vi "CameraControl.vi"(0 "Exposure Time":dbl=20011.0 min=61.0 max=16000000.0, 1 "Gain Selector":u32(ring)=1 items=["Sensor", "Digital"], 2 "Gain":dbl=1.0 min=1.0 max=4.0, 3 "Gain (Raw)":i64 min=0 max=384 step=1, 4 "Black Level Selector":u32(ring) items=["Analog"], 5 "Stop (F)":bool, 7 "error in":errorcluster, 8 "Black Level":dbl=240.0 min=0.0 max=511.0, 9 "Camera":string="S1104113") -> (6 "Lost Packet Count":u32, 20 "Image Out":T1(plugin-control), 21 "All Image Buffers Out":T1[](array[typedef]), 22 "Temp":dbl, 26 "Stopped":bool, 27 "error out":errorcluster)   [LabVIEW 2014]
doc: "Creates, and edits acquisitions using the NI Vision Acquisition Express VI.\n\nThe NI Vision Acquisition Wizard is launched by placing the Express VI on the block diagram. Select an acquisition source and configure an acquisition using NI-IMAQ, NI-IMAQdx, or simulate an acquisition by reading an AVI or image files from a folder. After an acquisition is configured, select controls and indicators to be able to programmatically set in LabVIEW. Double-click the Vision Acquisition Express VI to edit the acquisition.\n\nNote: Any images created by the Express VI need to be disposed after use. Use the IMAQ Dispose.vi to cleanup the images output by the Express VI when they are no longer needed."
uses:
  <vilib>/vision/Image Controls.llb/IMAQ Image.ctl
  <vilib>/vision/driver/IMAQdx.llb/IMAQdx Buffer Number Mode.ctl
  <vilib>/vision/driver/NI_Vision_Acquisition_Software.lvlib
  <resource>/objmgr/imaqdx.rc
panel:
  out "BufferCount":u32
  out "LostBufferCount":u32
  out "x != y? 6":bool
  out "x != y? 5":bool
  out "x != y? 4":bool
  out "x != y? 3":bool
  out "x != y? 2":bool
  out "x != y?":bool
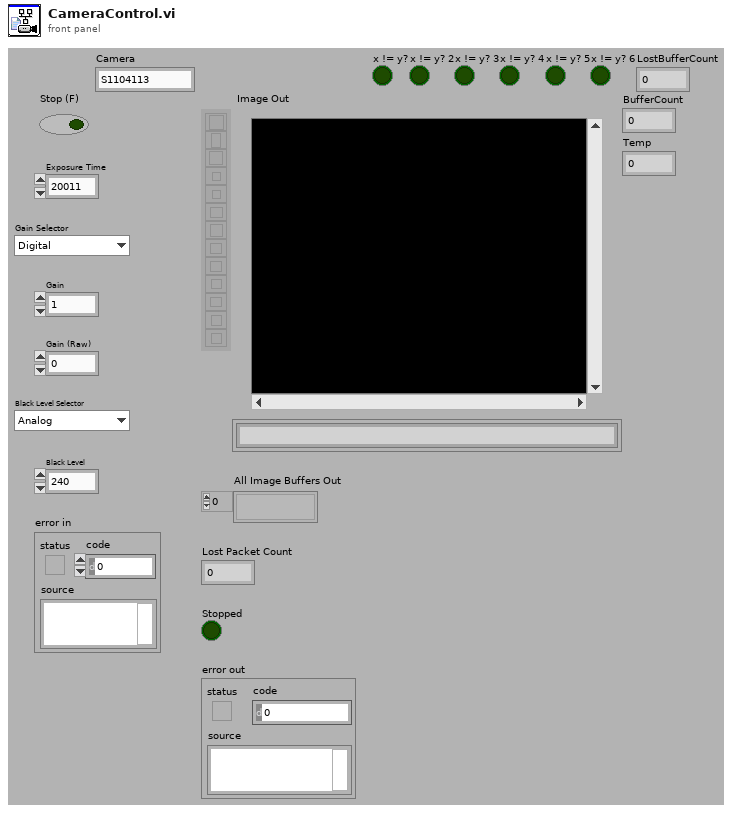
[diagram p1: front panel]
types:
  T1 = typedef "IMAQ Image.ctl" = refnum<image>
  T2 = typedef "NI_Vision_Acquisition_Software.lvlib/IMAQdx Buffer Number Mode.ctl" = enum32{"Next", "Last", "Buffer Number"}
  T3 = typedef "IMAQdx.ctl" = refnum<k21>
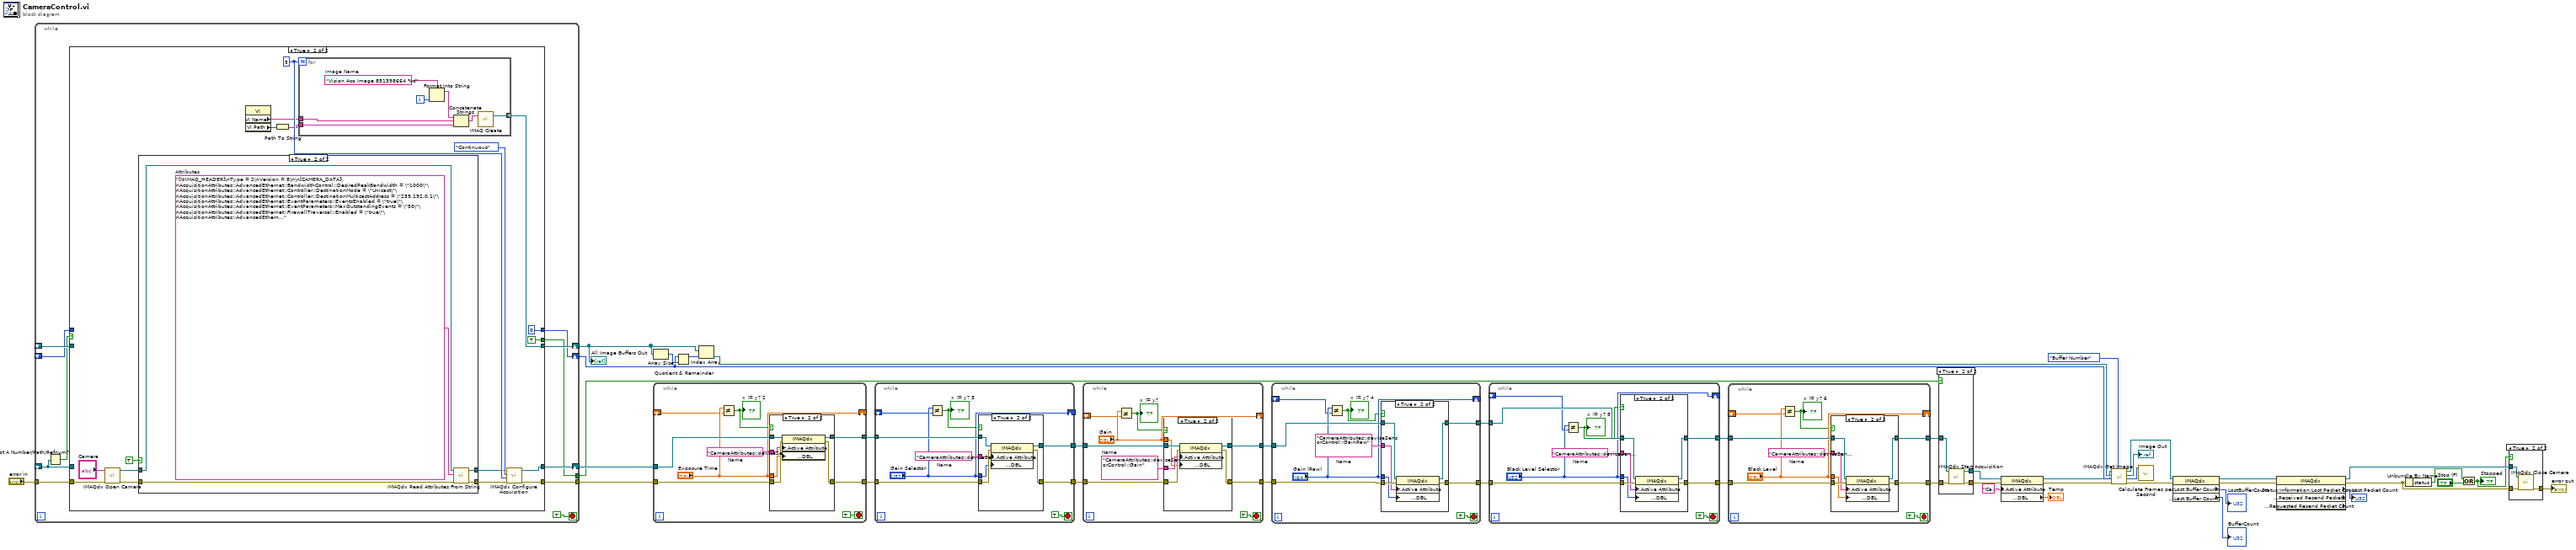
[diagram p0: block diagram]
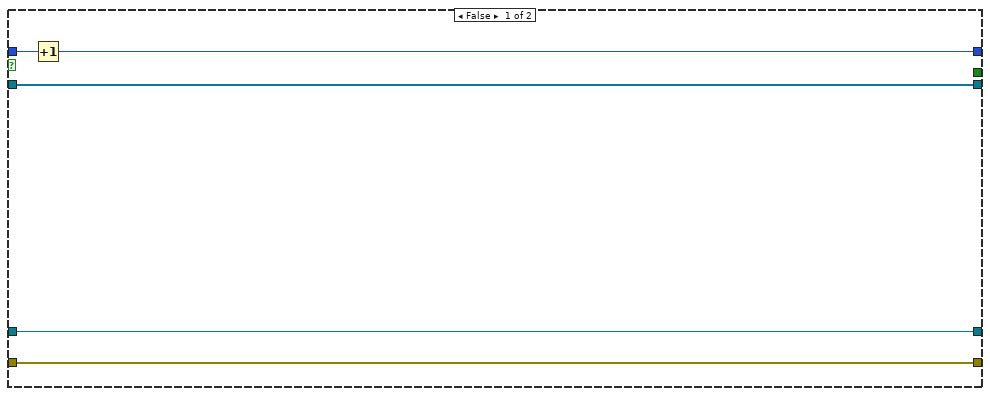
[diagram p10: hidden frame]
diagram:
  n1 = while {
    shift-right: [w54] -> w41
    shift-left: _ -> [w46]
    tunnel: [w53] -> w42
    tunnel: "error in" -> [w52]
    shift-right: [w50] -> w26
    shift-left: _ -> [w49]
    shift-right: [w48] -> w21
    shift-left: _ -> [w47]
    tunnel: [w44] -> w20
    stop <- TRUE stop-if-true
    n2 = Not A Number/Path/Refnum?(number/path/refnum=w46) -> (NaN/Path/Refnum?=w45:bool)
    n3 = case shown="True" w45 {
      tunnel: [w59 w60] -> w54
      tunnel: w46 -> [w59 _]
      tunnel: [w58 w75] -> w53
      tunnel: w52 -> [w58 w76]
      tunnel: [w57 w74] -> w50
      tunnel: w49 -> [w57 _]
      tunnel: [w55 0] -> w48
      tunnel: w47 -> [w56 _]
      tunnel: [_ TRUE] -> w44
      frame False {
        n4 = Increment(x=w56) -> (x+1=w55:i32)
      }
      frame True {
        w73 = u32 5 ("Number of Image Buffers")
        n5 = call <vilib>:"IMAQdx Open Camera.vi"("error in"=w76, "Session In"="Camera") -> ("error out"=w66:errorcluster, "Session Out"=w67:T3)  [unwired: 1 in, 7 out]
        n6 = case shown="True" TRUE ("Init Attributes") {
          tunnel: w67 -> [w78 w83]
          tunnel: w66 -> [w77 w82]
          tunnel: [w78 w79] -> w65
          tunnel: [w77 w80] -> w64
          frame False {
          }
          frame True {
            w81 = "[NIIMAQ_HEADER]\nType = 2\nVersion = 8\n\n[CAMERA_DATA]\nAcquisitionAttributes::AdvancedEthernet::BandwidthControl::DesiredPeakBandwidth = \"1000\"\nAcquisitionAttributes::AdvancedEthernet::Controller::DestinationMode = \"Unicast\"\nAcquisitionAttributes::AdvancedEthernet::Controller::DestinationMulticastAddress = \"239.192.0.1\"\nAcquisitionAttributes::AdvancedEthernet::EventParameters::EventsEnabled = \"true\"\nAcquisitionAttributes::AdvancedEthernet::EventParameters::MaxOutstandingEvents = \"50\"\nAcquisitionAttributes::AdvancedEthernet::FirewallTraversal::Enabled = \"true\"\nAcquisitionAttributes::AdvancedEthernet::FirewallTraversal::KeepAliveTime = \"30\"\nAcquisitionAttributes::AdvancedEthernet::ResendParameters::MaxResendsPerPacket = \"25\"\nAcquisitionAttributes::AdvancedEthernet::ResendParameters::MemoryWindowSize = \"1024\"\nAcquisitionAttributes::AdvancedEthernet::ResendParameters::MissingPacketTimeout = \"2\"\nAcquisitionAttributes::AdvancedEthernet::ResendParameters::NewPacketTimeout = \"100\"\nAcquisitionAttributes::AdvancedEthernet::ResendParameters::ResendBatchingPercentage = \"10\"\nAcquisitionAttributes::AdvancedEthernet::ResendParameters::ResendResponseTimeout = \"2\"\nAcquisitionAttributes::AdvancedEthernet::ResendParameters::ResendsEnabled = \"true\"\nAcquisitionAttributes::AdvancedEthernet::ResendParameters::ResendThresholdPercentage = \"5\"\nAcquisitionAttributes::AdvancedEthernet::ResendParameters::ResendTimerResolution = \"1\"\nAcquisitionAttributes::AdvancedEthernet::TestPacketParameters::MaxTestPacketRetries = \"1\"\nAcquisitionAttributes::AdvancedEthernet::TestPacketParameters::TestPacketEnabled = \"true\"\nAcquisitionAttributes::AdvancedEthernet::TestPacketParameters::TestPacketTimeout = \"250\"\nAcquisitionAttributes::AdvancedGenicam::CommandTimeout = \"100\"\nAcquisitionAttributes::Bayer::Algorithm = \"Bilinear\"\nAcquisitionAttributes::Bayer::GainB = \"1\"\nAcquisitionAttributes::Bayer::GainG = \"1\"\nAcquisitionAttributes::Bayer::GainR = \"1\"\nAcquisitionAttributes::Bayer::Pattern = \"Use hardware value\"\nAcquisitionAttributes::BitsPerPixel = \"Use hardware value\"\nAcquisitionAttributes::ChunkDataDecoding::ChunkDataDecodingEnabled = \"false\"\nAcquisitionAttributes::ChunkDataDecoding::MaximumChunkCopySize = \"64\"\nAcquisitionAttributes::IgnoreFirstFrame = \"false\"\nAcquisitionAttributes::ImageDecoderCopyMode = \"Auto\"\nAcquisitionAttributes::IncompleteBufferMode = \"Ignore\"\nAcquisitionAttributes::OutputImageType = \"Auto\"\nAcquisitionAttributes::OverwriteMode = \"Get Newest\"\nAcquisitionAttributes::PacketSize = \"1500\"\nAcquisitionAttributes::PixelSignedness = \"Use hardware value\"\nAcquisitionAttributes::ReceiveTimestampMode = \"None\"\nAcquisitionAttributes::ShiftPixelBits = \"false\"\nAcquisitionAttributes::SwapPixelBytes = \"false\"\nAcquisitionAttributes::Timeout = \"5000\"\nCameraAttributes::deviceCounterAndTimerControl::counterSelector = \"Counter 1\"\nCameraAttributes::deviceCounterAndTimerControl::counterMode = \"Off\"\nCameraAttributes::deviceCounterAndTimerControl::counterStartSource = \"Line 1\"\nCameraAttributes::deviceCounterAndTimerControl::counterStartLineActivation = \"Rising Edge\"\nCameraAttributes::deviceCounterAndTimerControl::counterIncrementalSource = \"Internal Clock\"\nCameraAttributes::deviceCounterAndTimerControl::counterResetSource = \"Reset Cmd\"\nCameraAttributes::deviceCounterAndTimerControl::counterDuration = \"1\"\nCameraAttributes::deviceCounterAndTimerControl::timerSelector = \"Timer 1\"\nCameraAttributes::deviceCounterAndTimerControl::timerMode = \"Off\"\nCameraAttributes::deviceCounterAndTimerControl::timerStartSource = \"Line 1\"\nCameraAttributes::deviceCounterAndTimerControl::timerStartLineActivation = \"Rising Edge\"\nCameraAttributes::deviceCounterAndTimerControl::timerDuration = \"1\"\nCameraAttributes::deviceSensorControl::AcquisitionFrameRate = \"30\"\nCameraAttributes::deviceSensorControl::BlackLevelSelector = \"Analog\"\nCameraAttributes::deviceSensorControl::BlackLevelRaw = \"240\"\nCameraAttributes::deviceSensorControl::exposureAlignment = \"Synchronous\"\nCameraAttributes::deviceSensorControl::ExposureMode = \"Timed\"\nCameraAttributes::deviceSensorControl::ExposureTime = \"20011\"\nCameraAttributes::deviceSensorControl::GainSelector = \"Sensor\"\nCameraAttributes::deviceSensorControl::Gain = \"1\"\nCameraAttributes::deviceSensorControl::GainSelector = \"Digital\"\nCameraAttributes::deviceSensorControl::Gain = \"1\"\nCameraAttributes::DigitalIOControl::LineSelector = \"Line 1\"\nCameraAttributes::DigitalIOControl::lineDetectionLevel = \"Threshold for TTL\"\nCameraAttributes::DigitalIOControl::LineInverter = \"false\"\nCameraAttributes::DigitalIOControl::lineDebouncingPeriod = \"0\"\nCameraAttributes::DigitalIOControl::LineSelector = \"Line 2\"\nCameraAttributes::DigitalIOControl::lineDetectionLevel = \"Threshold for TTL\"\nCameraAttributes::DigitalIOControl::LineInverter = \"false\"\nCameraAttributes::DigitalIOControl::lineDebouncingPeriod = \"0\"\nCameraAttributes::DigitalIOControl::LineSelector = \"Line 3\"\nCameraAttributes::DigitalIOControl::LineInverter = \"false\"\nCameraAttributes::DigitalIOControl::outputLineSource = \"Pulse On: Software Command\"\nCameraAttributes::DigitalIOControl::outputLinePulseDelay = \"0\"\nCameraAttributes::DigitalIOControl::outputLinePulseDuration = \"1\"\nCameraAttributes::DigitalIOControl::LineSelector = \"Line 4\"\nCameraAttributes::DigitalIOControl::LineInverter = \"false\"\nCameraAttributes::DigitalIOControl::outputLineSource = \"Pulse On: Software Command\"\nCameraAttributes::DigitalIOControl::outputLinePulseDelay = \"0\"\nCameraAttributes::DigitalIOControl::outputLinePulseDuration = \"1\"\nCameraAttributes::DigitalIOControl::LineSelector = \"Line 1\"\nCameraAttributes::DigitalIOControl::TriggerSelector = \"Single Frame Trigger(Start)\"\nCameraAttributes::DigitalIOControl::TriggerMode = \"Off\"\nCameraAttributes::DigitalIOControl::TriggerSelector = \"MultiFrame Trigger(Start)\"\nCameraAttributes::DigitalIOControl::TriggerMode = \"Off\"\nCameraAttributes::ImageFormatControl::Height = \"1200\"\nCameraAttributes::ImageFormatControl::OffsetX = \"0\"\nCameraAttributes::ImageFormatControl::OffsetY = \"0\"\nCameraAttributes::ImageFormatControl::PixelFormat = \"Monochrome 8-Bit\"\nCameraAttributes::ImageFormatControl::Width = \"1920\"\nCameraAttributes::TransportLayerControl::devicePacketResendBufferSize = \"24\"\n"  # Attributes
            n7 = call <vilib>:"IMAQdx Read Attributes From String.vi"("error in"=w82, "Attributes String In"=w81, "Session In"=w83) -> ("error out"=w80:errorcluster, "Session Out"=w79:T3)  [unwired: 7 out]
          }
        }
        n8 = property class="VI"() -> ("VI Name"=w69:string, "VI Path"=w70:path)  [unwired: 2 in, 2 out]
        n9 = Path To String(path=w70) -> (string=w68:string)
        n10 = for "For Loop_template0" {
          N: w73 -> [_]
          tunnel: [w90] -> w74 mode=indexing
          tunnel: w69 -> [w85]
          tunnel: w68 -> [w84]
          i -> [w89]
          w88 = "Vision Acq Image 851398664 %d"  # Image Name
          n11 = Format Into String(format string=w88, w89) -> (resulting string=w87:string)  [unwired: 2 in, 1 out]
          n12 = Concatenate Strings(w87, w85, w84) -> (w86:string)
          n13 = call "IMAQ Create"("Image Name"=w86) -> ("New Image"=w90:T1)  [unwired: 3 in, 2 out]
        }
        n14 = call <vilib>:"IMAQdx Configure Acquisition.vi"("error in"=w64, "Number of Buffers"=w73, "Continuous?"=enum32{"One Shot", "Continuous"}."Continuous" ("Mode"), "Session In"=w65) -> ("error out"=w75:errorcluster, "Session Out"=w60:T3)  [unwired: 6 out]
      }
    }
  }
  "All Image Buffers Out" <- w26
  n15 = Array Size(array=w26) -> (size(s)=w27:i32)
  n16 = while {
    tunnel: w42 -> [w99]
    tunnel: [w98] -> w39
    tunnel: w41 -> [w97]
    tunnel: [w96] -> w40
    shift-right: ["Exposure Time"] -> _
    shift-left: _ -> [w92]
    stop <- TRUE stop-if-true
    w95 = "CameraAttributes::deviceSensorControl::ExposureTime"  # Name
    n17 = Not Equal?(x="Exposure Time", y=w92) -> (x != y?=w91:bool)
    "x != y? 2" <- w91
    n18 = case shown="True" w91 {
      tunnel: w99 -> [w100 w107]
      tunnel: [w101 w106] -> w98
      tunnel: w97 -> [w101 w105]
      tunnel: [w100 w104] -> w96
      tunnel: w95 -> [_ w103]
      tunnel: "Exposure Time" -> [_ w102]
      frame False {
      }
      frame True {
        n19 = property class="IMAQdx"(reference=w105, error in=w107, "Camera Attributes:Active Attribute"=w103, "Camera Attributes:Value:DBL"=w102) -> (reference out=w106:T3, error out=w104:errorcluster)
      }
    }
  }
  n20 = Quotient & Remainder(x=w21, y=w27) -> (x-y*floor(x/y)=w25:i32)  [unwired: 1 out]
  n21 = Index Array(array=w26, index=w25) -> (element=w24:T1)
  n22 = while {
    tunnel: w40 -> [w116]
    tunnel: [w115] -> w37
    tunnel: w39 -> [w114]
    tunnel: [w113] -> w38
    shift-right: ["Gain Selector"] -> _
    shift-left: _ -> [w109]
    stop <- TRUE stop-if-true
    w112 = "CameraAttributes::deviceSensorControl::GainSelector"  # Name
    n23 = Not Equal?(x="Gain Selector", y=w109) -> (x != y?=w108:bool)
    "x != y? 3" <- w108
    n24 = case shown="True" w108 {
      tunnel: w116 -> [w117 w124]
      tunnel: [w118 w123] -> w115
      tunnel: w114 -> [w118 w122]
      tunnel: [w117 w121] -> w113
      tunnel: w112 -> [_ w120]
      tunnel: "Gain Selector" -> [_ w119]
      frame False {
      }
      frame True {
        n25 = property class="IMAQdx"(reference=w122, error in=w124, "Camera Attributes:Active Attribute"=w120, "Camera Attributes:Value:DBL"=w119) -> (reference out=w123:T3, error out=w121:errorcluster)
      }
    }
  }
  n26 = while {
    tunnel: w38 -> [w133]
    tunnel: [w132] -> w35
    tunnel: w37 -> [w131]
    tunnel: [w130] -> w36
    shift-right: ["Gain"] -> _
    shift-left: _ -> [w126]
    stop <- TRUE stop-if-true
    w129 = "CameraAttributes::deviceSensorControl::Gain"  # Name
    n27 = Not Equal?(x="Gain", y=w126) -> (x != y?=w125:bool)
    "x != y?" <- w125
    n28 = case shown="True" w125 {
      tunnel: w133 -> [w134 w141]
      tunnel: [w135 w140] -> w132
      tunnel: w131 -> [w135 w139]
      tunnel: [w134 w138] -> w130
      tunnel: w129 -> [_ w137]
      tunnel: "Gain" -> [_ w136]
      frame False {
      }
      frame True {
        n29 = property class="IMAQdx"(reference=w139, error in=w141, "Camera Attributes:Active Attribute"=w137, "Camera Attributes:Value:DBL"=w136) -> (reference out=w140:T3, error out=w138:errorcluster)
      }
    }
  }
  n30 = while {
    tunnel: w36 -> [w150]
    tunnel: [w149] -> w33
    tunnel: w35 -> [w148]
    tunnel: [w147] -> w34
    shift-right: ["Gain (Raw)"] -> _
    shift-left: _ -> [w143]
    stop <- TRUE stop-if-true
    w146 = "CameraAttributes::deviceSensorControl::GainRaw"  # Name
    n31 = Not Equal?(x="Gain (Raw)", y=w143) -> (x != y?=w142:bool)
    "x != y? 4" <- w142
    n32 = case shown="True" w142 {
      tunnel: w150 -> [w151 w158]
      tunnel: [w152 w157] -> w149
      tunnel: w148 -> [w152 w156]
      tunnel: [w151 w155] -> w147
      tunnel: w146 -> [_ w154]
      tunnel: "Gain (Raw)" -> [_ w153]
      frame False {
      }
      frame True {
        n33 = property class="IMAQdx"(reference=w156, error in=w158, "Camera Attributes:Active Attribute"=w154, "Camera Attributes:Value:DBL"=w153) -> (reference out=w157:T3, error out=w155:errorcluster)
      }
    }
  }
  n34 = while {
    tunnel: w34 -> [w167]
    tunnel: [w166] -> w7
    tunnel: w33 -> [w165]
    tunnel: [w164] -> w32
    shift-right: ["Black Level Selector"] -> _
    shift-left: _ -> [w160]
    stop <- TRUE stop-if-true
    w163 = "CameraAttributes::deviceSensorControl::BlackLevelSelector"  # Name
    n35 = Not Equal?(x="Black Level Selector", y=w160) -> (x != y?=w159:bool)
    "x != y? 5" <- w159
    n36 = case shown="True" w159 {
      tunnel: w167 -> [w168 w175]
      tunnel: [w169 w174] -> w166
      tunnel: w165 -> [w169 w173]
      tunnel: [w168 w172] -> w164
      tunnel: w163 -> [_ w171]
      tunnel: "Black Level Selector" -> [_ w170]
      frame False {
      }
      frame True {
        n37 = property class="IMAQdx"(reference=w173, error in=w175, "Camera Attributes:Active Attribute"=w171, "Camera Attributes:Value:DBL"=w170) -> (reference out=w174:T3, error out=w172:errorcluster)
      }
    }
  }
  n38 = while {
    tunnel: w32 -> [w184]
    tunnel: [w183] -> w22
    tunnel: w7 -> [w182]
    tunnel: [w181] -> w31
    shift-right: ["Black Level"] -> _
    shift-left: _ -> [w177]
    stop <- TRUE stop-if-true
    w180 = "CameraAttributes::deviceSensorControl::BlackLevel"  # Name
    n39 = Not Equal?(x="Black Level", y=w177) -> (x != y?=w176:bool)
    "x != y? 6" <- w176
    n40 = case shown="True" w176 {
      tunnel: w184 -> [w185 w192]
      tunnel: [w186 w191] -> w183
      tunnel: w182 -> [w186 w190]
      tunnel: [w185 w189] -> w181
      tunnel: w180 -> [_ w188]
      tunnel: "Black Level" -> [_ w187]
      frame False {
      }
      frame True {
        n41 = property class="IMAQdx"(reference=w190, error in=w192, "Camera Attributes:Active Attribute"=w188, "Camera Attributes:Value:DBL"=w187) -> (reference out=w191:T3, error out=w189:errorcluster)
      }
    }
  }
  n42 = case shown="True" w20 {
    tunnel: w22 -> [w194 w198]
    tunnel: w31 -> [w193 w197]
    tunnel: [w193 w195] -> w2
    tunnel: [w194 w196] -> w4
    frame False {
    }
    frame True {
      n43 = call <vilib>:"IMAQdx Start Acquisition.vi"("error in"=w197, "Session In"=w198) -> ("error out"=w195:errorcluster, "Session Out"=w196:T3)  [unwired: 8 out]
    }
  }
  n44 = property class="IMAQdx"(reference=w4, error in=w2, "Camera Attributes:Active Attribute"="CameraAttributes::deviceInformation::DeviceTemperature") -> (reference out=w3:T3, error out=w1:errorcluster, "Camera Attributes:Value:DBL"=→"Temp":dbl)
  n45 = call <vilib>:"IMAQdx Get Image.vi"("Buffer Number Mode (Next)"=IMAQdx_Buffer_Number_Mode."Buffer Number", "error in"=w1, "Buffer Number In"=w21, "Image In"=w24, "Session In"=w3) -> ("error out"=w29:errorcluster, "Buffer Number Out"=w19:u32, "Image Out"=→"Image Out":T1, "Session Out"=w30:T3)  [unwired: 3 out]
  n46 = call <vilib>:"Calculate Frames per Second.vi"("Buffer Number"=w19) -> ()  [unwired: 2 in, 9 out]
  n47 = property class="IMAQdx"(reference=w30, error in=w29) -> (reference out=w17:T3, error out=w23:errorcluster, "Status Information:Lost Buffer Count"=→"LostBufferCount":u32, "Status Information:Last Buffer Count"=→"BufferCount":u32)
  n48 = property class="IMAQdx" props=["Status Information:Lost Packet Count", "Status Information:Received Resend Packets", "Status Information:Requested Resend Packet Count"](reference=w17, error in=w23) -> (reference out=w14:T3, error out=w16:errorcluster, "Status Information:Lost Packet Count"=→"Lost Packet Count":u32)  [unwired: 2 out]
  n49 = Unbundle By Name(w16) -> ("status"=w10:bool)
  n50 = Or(x=w10, y="Stop (F)") -> (x .or. y?=w11:bool)
  "Stopped" <- w11
  n51 = case "Case Structure_template1" shown="True" w11 {
    tunnel: [w199 w201] -> w13
    tunnel: w16 -> [w199 w202]
    tunnel: w14 -> [_ w200]
    frame False {
    }
    frame True {
      n52 = call <vilib>:"IMAQdx Close Camera.vi"("error in"=w202, "Session In"=w200) -> ("error out"=w201:errorcluster)  [unwired: 9 out]
    }
  }
  "error out" <- w13
